vi "init gamepad.vi"() -> (0 "device ID":refnum<k1>, 1 "Joystick found":bool)   [LabVIEW 2012]
uses:
  <vilib>/Utility/inputDevices.llb/joystickAcquire.vi
  <vilib>/Utility/inputDevices.llb/closeJoystick.vi
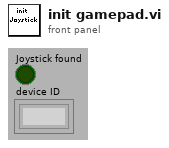
[diagram p1: front panel]
types:
  T1 = cluster{"axes total":u32, "buttons total":u32, "pov total":u32, "device name":string}[]
  T2 = cluster{"button 1":bool, "button 2":bool, "button 3":bool, "button 4":bool, "button 5":bool, "button 6":bool, "button 7":bool, "button 8":bool, "button 9":bool, "button 10":bool, "button 11":bool, "button 12":bool, "button 13":bool, "button 14":bool, "button 15":bool, "button 16":bool, "button 17":bool, "button 18":bool, "button 19":bool, "button 20":bool, "button 21":bool, "button 22":bool, "button 23":bool, "button 24":bool, "button 25":bool, "button 26":bool, "button 27":bool, "button 28":bool, "button 29":bool, "button 30":bool, "button 31":bool, "button 32":bool}
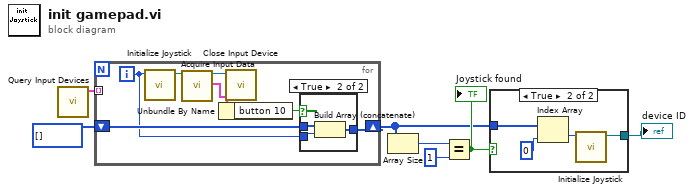
[diagram p0: block diagram]
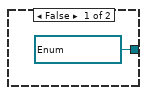
[diagram p2: hidden frame]
diagram:
  n1 = call <vilib>:"Query Input Devices.vi"() -> ("joystick info"=w1:T1)  [unwired: 1 in, 10 out]
  n2 = for {
    shift-right: [w10] -> w3
    shift-left: i32[] [] ("appended array") -> [w11]
    tunnel: w1 -> [_] mode=indexing
    i -> [w9]
    n3 = call <vilib>:"Initialize Joystick.vi"("device index"=w9) -> ("device ID"=w14:refnum<k1>)  [unwired: 1 in, 9 out]
    n4 = call-poly <vilib>:"Acquire Input Data.vi"("device ID"=w14) -> ("device ID"=w13:refnum<k1>, "button info"=w12:T2)  [unwired: 1 in, 16 out]
    n5 = Unbundle By Name(w12) -> ("button 10"=w8:bool)
    n6 = call-poly <vilib>:"Close Input Device.vi"("device ID"=w13) -> ()  [unwired: 1 in, 9 out]
    n7 = case shown="True" w8 {
      tunnel: w11 -> [w15 w16]
      tunnel: [w15 w17] -> w10
      tunnel: w9 -> [_ w18]
      frame False {
      }
      frame True {
        n8 = Build Array (concatenate)(w16, w18) -> (w17:i32[])
      }
    }
  }
  n9 = Array Size(array=w3) -> (size(s)=w5:i32)
  n10 = Equal?(x=w5, y=1) -> (x = y?=w4:bool)
  "Joystick found" <- w4
  n11 = case shown="True" w4 {
    tunnel: w3 -> [_ w23]
    tunnel: [w19 w20] -> w2
    frame False {
      w19 = refnum<k1> refnum items=["JOYSTICK"] ("device ID")
    }
    frame True {
      n12 = Index Array(array=w23, index=0) -> (element=w21:i32)
      n13 = call <vilib>:"Initialize Joystick.vi"("device index"=w21) -> ("device ID"=w20:refnum<k1>)  [unwired: 1 in, 9 out]
    }
  }
  "device ID" <- w2
